vi "AccelFilters.vi"(8 "error in":errorcluster, 11 "Cutoff Frequncies":T1[](array[typedef]) {"HP Passband" min=1.0 step=1.0 format="%#.4f"; "LP Stopband" min=1.0 step=1.0 format="%#.4f"; "HP Stopband" min=1.0 step=1.0 format="%#.4f"; "LP Passband" min=1.0 step=1.0 format="%#.4f"}) -> (0 "error out":errorcluster)   [LabVIEW 2018, in "Vibration.lvlib"]
doc: "This subVI enqueues the named action in to the communications queue along with the input data."
uses:
  Vibration.lvlib
  Modules/Testing UI 3/Private Controls/Cutoff Frequency.ctl
  Private Controls/Module Data.ctl
  Private Controls/Module Action.ctl
  Modules/Testing UI 3/Testing UI 3.lvlib
panel:
  # "Highpass Cutoff Frequency"
  # "Lowpass Cutoff Frequency"
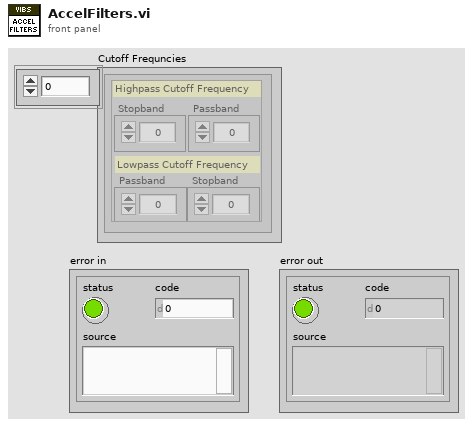
[diagram p1: front panel]
types:
  T1 = typedef "Testing UI 3.lvlib/Cutoff Frequency.ctl" = cluster{"LP Passband":dbl, "HP Stopband":dbl, "LP Stopband":dbl, "HP Passband":dbl}
  T2 = typedef "Vibration.lvlib/Module Data.ctl" = cluster{"Data":variant, "Action":T3}
  T3 = typedef "Vibration.lvlib/Module Action.ctl" = enum16{"Init", "Waterfall Select", "Read", "Accel Sensitivities", "Filters", "Error"}
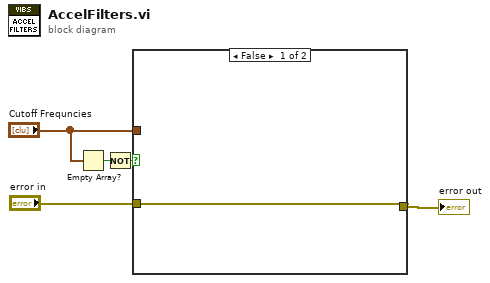
[diagram p0: block diagram]
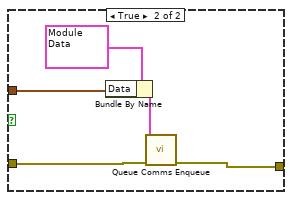
[diagram p2: hidden frame]
diagram:
  n1 = Empty Array?(array="Cutoff Frequncies") -> (empty?=w2:bool)
  n2 = Not(x=w2) -> (.not. x?=w1:bool)
  n3 = case shown="False" w1 {
    tunnel: [w6 w11] -> w5
    tunnel: "error in" -> [w6 w10]
    tunnel: "Cutoff Frequncies" -> [_ w7]
    frame False {
    }
    frame True {
      n4 = Bundle By Name(cluster=T2 {"Data"=variant, "Action"=enum."Filters"} ("element"), "Data"=w7) -> (w8:T2)
      n5 = call "Queue Comms Enqueue.vi"("error in (no error)"=w10, "element"=w8) -> ("error out"=w11:errorcluster)  [unwired: 9 in]
    }
  }
  "error out" <- w5
